vi "IMS Send Command_mod.vi"() -> (0 "error out":errorcluster, 2 "read buffer":string, 3 "VISA resource name out":refnum<visa-resource-name>)   [LabVIEW 2009]
uses:
  <vilib>/Instr/_visa.llb/VISA Configure Serial Port (Instr).vi
panel:
  in  "String":string
  out "Serial Settings:Number of Bytes at Serial Port":u32
  in  "baud rate (9600)":u32=9600
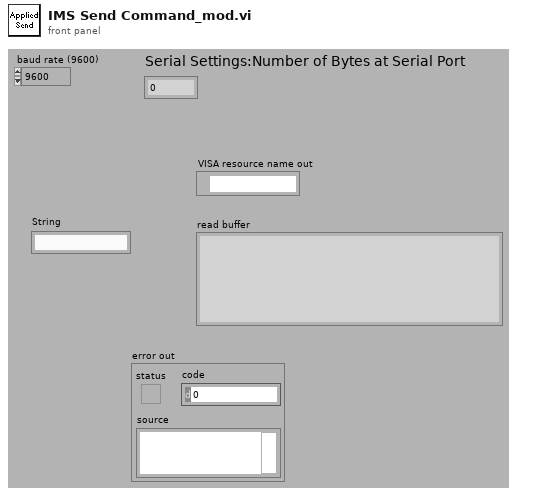
[diagram p1: front panel]
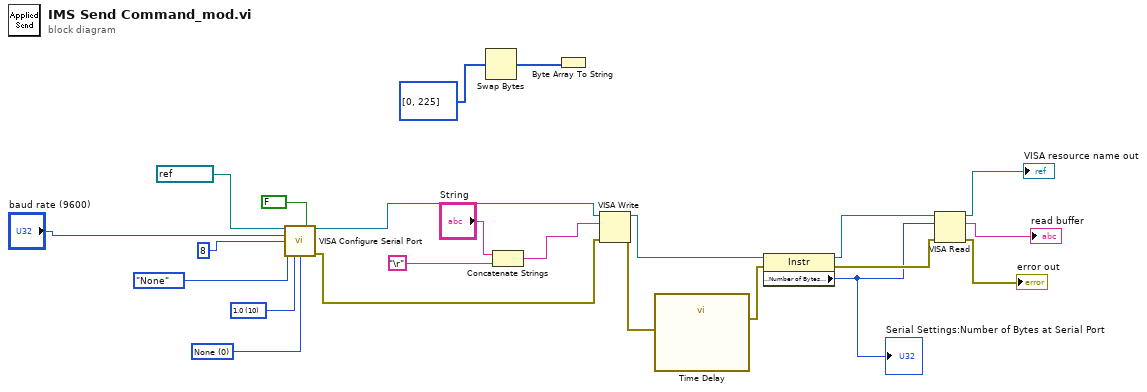
[diagram p0: block diagram]
diagram:
  w17 = u16 0 items=["None", "XON/XOFF", "RTS/CTS", "XON/XOFF & RTS/CTS", "DTR/DSR", "XON/XOFF & DTR/DSR"] ("flow control (0:none)")
  w19 = u16 10 items=["1.0"=10, "1.5"=15, "2.0"=20] ("stop bits (10: 1 bit)")
  n1 = call-poly "VISA Configure Serial Port"("VISA resource name"=refnum<visa-resource-name> "COM1", "Enable Termination\nChar (T)"=FALSE ("Enable Termination\nChar (T)"), "baud rate (9600)"="baud rate (9600)", "data bits (8)"=u16 8, "parity (0:none)"=enum16{"None", "Odd", "Even", "Mark", "Space"}."None", "stop bits (10: 1 bit)"=w19, "flow control (0:none)"=w17) -> ("VISA resource name out"=w16:refnum<visa-resource-name>, "error out"=w15:errorcluster)  [unwired: 7 in]
  n2 = Swap Bytes(anything=u8[] [0, 225] ("unsigned byte array")) -> (byte swapped=w5:u8[])
  n3 = Concatenate Strings("String", "\r") -> (w4:string)
  n4 = Byte Array To String(unsigned byte array=w5) -> ()  [unwired: 1 out]
  n5 = VISA Write(VISA resource name=w16, write buffer=w4, error in (no error)=w15) -> (VISA resource name out=w12:refnum<visa-resource-name>, error out=w9:errorcluster)  [unwired: 1 out]
  n6 = call "Time Delay"("error in (no error)"=w9) -> ("error out"=w8:errorcluster)  [unwired: 10 in]
  n7 = property class="Instr"(reference=w12, error in=w8) -> (reference out=w11:refnum<visa-resource-name>, error out=w10:errorcluster, "Serial Settings:Number of Bytes at Serial Port"=w1:u32)
  "Serial Settings:Number of Bytes at Serial Port" <- w1
  n8 = VISA Read(VISA resource name=w11, byte count=w1, error in (no error)=w10) -> (VISA resource name out=→"VISA resource name out":refnum<visa-resource-name>, read buffer=→"read buffer":string, error out=→"error out":errorcluster)  [unwired: 1 out]
